vi "PROJECT_Evaluate Default Menu Selection.vi"(8 "error in":errorcluster, 10 "ItemPath":string, 11 "ItemTag":string) -> (0 "error out":errorcluster)   [LabVIEW 2022 SP3, in "Project.lvlib"]
doc: "____\nHAMPEL SOFTWARE ENGINEERING v2.6.0 (2023-12-19 10:54)"
uses:
  Project.lvlib
  <vilib>/Hampel Software Engineering/HSE Logger/hse-logger.lvlib
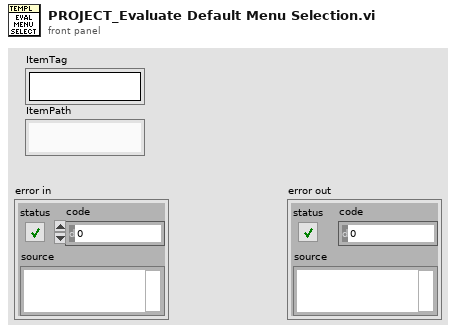
[diagram p1: front panel]
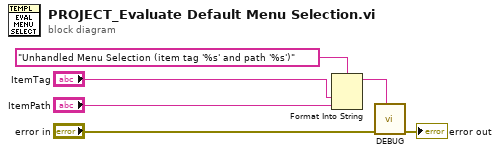
[diagram p0: block diagram]
diagram:
  n1 = Format Into String(format string="Unhandled Menu Selection (item tag '%s' and path '%s')", "ItemTag", "ItemPath") -> (resulting string=w1:string)  [unwired: 2 in, 1 out]
  n2 = call <vilib>:"DEBUG.vi"("Message"=w1, "error in"="error in") -> ("error out"=→"error out":errorcluster)  [unwired: 9 in]
